vi "setupScene.vi"(11 "Model File Path":path=path "K:/Google_Drive/3d_Parts/Parts_for_printer/forLabview/yArm.stl") -> (3 "reference out":refnum<vi>)   [LabVIEW 2015]
uses:
  <vilib>/Utility/miscctls.llb/LVRGBAColorTypeDef.ctl
  <vilib>/Utility/miscctls.llb/LV3DPointTypeDef.ctl
  <vilib>/picture/3D Picture Control/Object/Create Object (name).vi
  <vilib>/picture/3D Picture Control/NI_3D Picture Control.lvlib
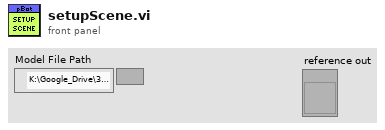
[diagram p1: front panel]
types:
  T1 = enum16{"Inherit Value", "Points", "Wireframe", "Polygons"}
  T2 = typedef "LVRGBAColorTypeDef.ctl" = cluster{"Red":sgl, "Green":sgl, "Blue":sgl, "Alpha":sgl}
  T3 = typedef "LV3DPointTypeDef.ctl" = cluster{"X":sgl, "Y":sgl, "Z":sgl}
  T4 = enum16{"Inherit Value", "Counterclockwise", "Clockwise"}
  T5 = enum16{"Inherit Value", "No Culling", "Cull Back Face", "Cull Front Face", "Cull Both Faces"}
  T6 = enum16{"Normal Bin", "Opaque Bin", "Transparent Bin"}
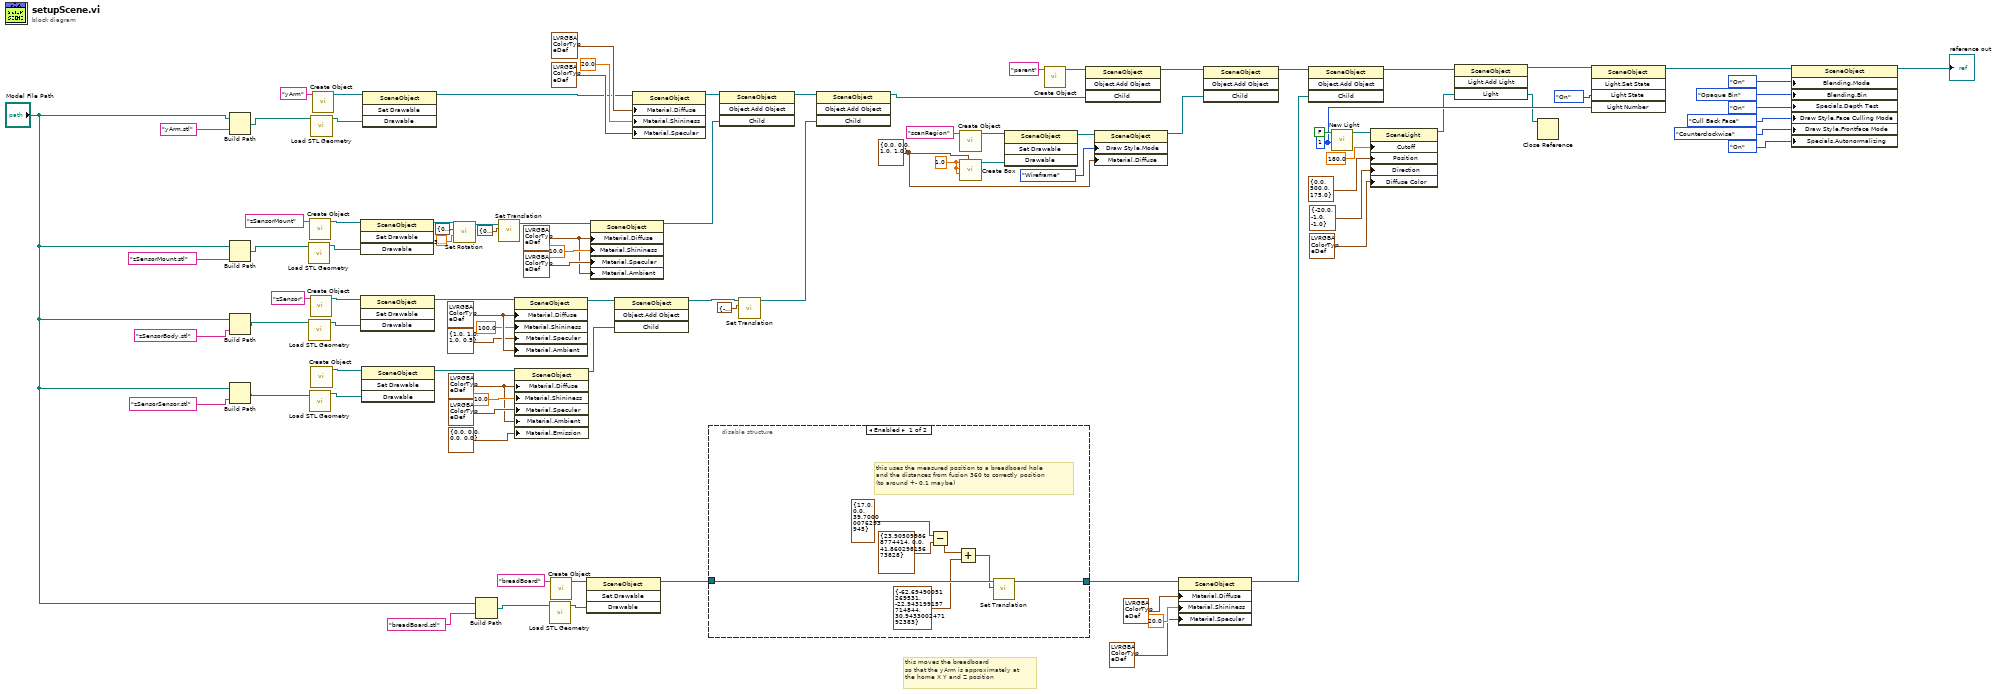
[diagram p0: block diagram]
diagram:
  w4 = T2 {"Red"=0.0, "Green"=0.0, "Blue"=1.0, "Alpha"=1.0} ("Material:Diffuse")
  w8 = sgl 1.0 ("Length X")
  w32 = T2 {"Red"=0.8, "Green"=0.5, "Blue"=0.2, "Alpha"=1.0} ("Material:Specular")
  w43 = T2 {"Red"=0.6, "Green"=0.6, "Blue"=0.6, "Alpha"=1.0} ("Material:Specular")
  w44 = T2 {"Red"=0.7, "Green"=0.7, "Blue"=0.0, "Alpha"=0.9} ("Material:Specular")
  w69 = 1 ("Light Number")
  # "this moves the breadboard\nso that the yArm is approximately at\nthe home X Y and Z position"
  n1 = Build Path(base path="Model File Path", name or relative path="yArm.stl" ("Model File")) -> (appended path=w22:path)
  n2 = Build Path(base path="Model File Path", name or relative path="zSensorMount.stl" ("Model File")) -> (appended path=w16:path)
  n3 = Build Path(base path="Model File Path", name or relative path="zSensorBody.stl" ("Model File")) -> (appended path=w17:path)
  n4 = Build Path(base path="Model File Path", name or relative path="zSensorSensor.stl" ("Model File")) -> (appended path=w18:path)
  n5 = call <vilib>:"Load STL Geometry.vi"("Model File"=w16) -> ("New Mesh Refnum"=w54:refnum<vi>)  [unwired: 9 in, 1 out]
  n6 = call <vilib>:"Load STL Geometry.vi"("Model File"=w17) -> ("New Mesh Refnum"=w40:refnum<vi>)  [unwired: 9 in, 1 out]
  n7 = call-poly <vilib>:"Create Object.vi"("Name"="zSensorMount") -> ("Scene:New Object"=w55:refnum<vi>)  [unwired: 9 in, 1 out]
  n8 = call <vilib>:"Load STL Geometry.vi"("Model File"=w18) -> ("New Mesh Refnum"=w35:refnum<vi>)  [unwired: 9 in, 1 out]
  n9 = call-poly <vilib>:"Create Object.vi"("Name"="zSensor") -> ("Scene:New Object"=w39:refnum<vi>)  [unwired: 9 in, 1 out]
  n10 = call <vilib>:"Load STL Geometry.vi"("Model File"=w22) -> ("New Mesh Refnum"=w93:refnum<vi>)  [unwired: 9 in, 1 out]
  n11 = call-poly <vilib>:"Create Object.vi"() -> ("Scene:New Object"=w36:refnum<vi>)  [unwired: 10 in, 1 out]
  n12 = call-poly <vilib>:"Create Object.vi"("Name"="yArm") -> ("Scene:New Object"=w94:refnum<vi>)  [unwired: 9 in, 1 out]
  n13 = invoke class="SceneObject" method="Set Drawable"(reference=w55, "Drawable"=w54) -> (reference out=w48:refnum<vi>)  [unwired: 2 in, 3 out]
  n14 = invoke class="SceneObject" method="Set Drawable"(reference=w39, "Drawable"=w40) -> (reference out=w30:refnum<vi>)  [unwired: 2 in, 3 out]
  n15 = invoke class="SceneObject" method="Set Drawable"(reference=w36, "Drawable"=w35) -> (reference out=w29:refnum<vi>)  [unwired: 2 in, 3 out]
  n16 = invoke class="SceneObject" method="Set Drawable"(reference=w94, "Drawable"=w93) -> (reference out=w12:refnum<vi>)  [unwired: 2 in, 3 out]
  n17 = call <vilib>:"Set Rotation.vi"("Angle"=3.141592653589793, "Axis"=cluster{"X":sgl, "Y":sgl, "Z":sgl} {"X"=0.0, "Y"=1.0, "Z"=0.0}, "Scene Object"=w48) -> ("Rotated Scene Object"=w45:refnum<vi>)  [unwired: 7 in, 1 out]
  n18 = Build Path(base path="Model File Path", name or relative path="breadBoard.stl" ("Model File")) -> (appended path=w15:path)
  n19 = call <vilib>:"Set Translation.vi"("Translation"=cluster{"X":sgl, "Y":sgl, "Z":sgl} {"X"=0.0, "Y"=4.7625, "Z"=-5.0}, "Scene Object"=w45) -> ("Translated Object"=w51:refnum<vi>)  [unwired: 8 in, 1 out]
  n20 = property class="SceneObject"(reference=w30, "Material.Diffuse"=w43, "Material.Shininess"=sgl 100.0 ("Material:Shininess"), "Material.Specular"=T2 {"Red"=1.0, "Green"=1.0, "Blue"=1.0, "Alpha"=0.5} ("Material:Specular"), "Material.Ambient"=w43) -> (reference out=w37:refnum<vi>)  [unwired: 1 in, 1 out]
  n21 = property class="SceneObject"(reference=w29, "Material.Diffuse"=w32, "Material.Shininess"=sgl 10.0 ("Material:Shininess"), "Material.Specular"=T2 {"Red"=0.5, "Green"=0.2, "Blue"=0.0, "Alpha"=0.5} ("Material:Specular"), "Material.Ambient"=w32, "Material.Emission"=T2 {"Red"=0.0, "Green"=0.0, "Blue"=0.0, "Alpha"=0.0} ("Material:Emission")) -> (reference out=w28:refnum<vi>)  [unwired: 1 in, 1 out]
  n22 = call <vilib>:"Load STL Geometry.vi"("Model File"=w15) -> ("New Mesh Refnum"=w87:refnum<vi>)  [unwired: 9 in, 1 out]
  n23 = call-poly <vilib>:"Create Object.vi"("Name"="breadBoard") -> ("Scene:New Object"=w86:refnum<vi>)  [unwired: 9 in, 1 out]
  n24 = invoke class="SceneObject" method="Set Drawable"(reference=w86, "Drawable"=w87) -> (reference out=w85:refnum<vi>)  [unwired: 2 in, 3 out]
  n25 = property class="SceneObject"(reference=w51, "Material.Diffuse"=w44, "Material.Shininess"=sgl 10.0 ("Material:Shininess"), "Material.Specular"=T2 {"Red"=0.6, "Green"=0.6, "Blue"=0.2, "Alpha"=0.5} ("Material:Specular"), "Material.Ambient"=w44) -> (reference out=w49:refnum<vi>)  [unwired: 1 in, 1 out]
  n26 = invoke class="SceneObject" method="Object.Add Object"(reference=w37, "Child"=w28) -> (reference out=w27:refnum<vi>)  [unwired: 2 in, 3 out]
  n27 = property class="SceneObject"(reference=w12, "Material.Diffuse"=T2 {"Red"=0.3, "Green"=0.3, "Blue"=0.3, "Alpha"=1.0} ("Material:Diffuse"), "Material.Shininess"=sgl 20.0 ("Material:Shininess"), "Material.Specular"=T2 {"Red"=0.4, "Green"=0.4, "Blue"=0.4, "Alpha"=0.8} ("Material:Specular")) -> (reference out=w50:refnum<vi>)  [unwired: 1 in, 1 out]
  n28 = disable-structure shown="Enabled" {
    disable-tunnel: w85 -> [w101 w102]
    disable-tunnel: [w100 w102] -> w74
    frame Enabled {
      # "this uses the measured position to a breadboard hole\nand the distances from fusion 360 to correctly position\n(to around +- 0.1 maybe)"
      n29 = Subtract(x=cluster{"X":sgl, "Y":sgl, "Z":sgl} {"X"=17.0, "Y"=0.0, "Z"=39.7} ("Translation"), y=cluster{"X":sgl, "Y":sgl, "Z":sgl} {"X"=23.9051, "Y"=0.0, "Z"=41.8603} ("Translation")) -> (x-y=w96:cluster{"X":sgl, "Y":sgl, "Z":sgl})
      n30 = Add(x=w96, y=cluster{"X":sgl, "Y":sgl, "Z":sgl} {"X"=-62.6949, "Y"=-22.9432, "Z"=30.9433} ("Translation")) -> (x+y=w95:cluster{"X":sgl, "Y":sgl, "Z":sgl})
      n31 = call <vilib>:"Set Translation.vi"("Translation"=w95, "Scene Object"=w101) -> ("Translated Object"=w100:refnum<vi>)  [unwired: 8 in, 1 out]
    }
    frame Disabled {
    }
  }
  n32 = invoke class="SceneObject" method="Object.Add Object"(reference=w50, "Child"=w49) -> (reference out=w26:refnum<vi>)  [unwired: 2 in, 3 out]
  n33 = call <vilib>:"Set Translation.vi"("Translation"=cluster{"X":sgl, "Y":sgl, "Z":sgl} {"X"=-15.08, "Y"=1.0, "Z"=-5.0}, "Scene Object"=w27) -> ("Translated Object"=w25:refnum<vi>)  [unwired: 8 in, 1 out]
  n34 = invoke class="SceneObject" method="Object.Add Object"(reference=w26, "Child"=w25) -> (reference out=w11:refnum<vi>)  [unwired: 2 in, 3 out]
  n35 = call-poly <vilib>:"Create Object.vi"("Name"="scanRegion") -> ("Scene:New Object"=w6:refnum<vi>)  [unwired: 9 in, 1 out]
  n36 = call <vilib>:"Create Box.vi"("Color"=w4, "Length Z"=w8, "Length Y"=w8, "Length X"=w8) -> ("New Box Refnum"=w1:refnum<vi>)  [unwired: 6 in, 1 out]
  n37 = invoke class="SceneObject" method="Set Drawable"(reference=w6, "Drawable"=w1) -> (reference out=w5:refnum<vi>)  [unwired: 2 in, 3 out]
  n38 = call-poly <vilib>:"Create Object.vi"("Name"="parent") -> ("Scene:New Object"=w91:refnum<vi>)  [unwired: 9 in, 1 out]
  n39 = invoke class="SceneObject" method="Object.Add Object"(reference=w91, "Child"=w11) -> (reference out=w10:refnum<vi>)  [unwired: 2 in, 3 out]
  n40 = property class="SceneObject"(reference=w5, "Draw Style.Mode"=T1."Wireframe" ("Draw Style:Mode"), "Material.Diffuse"=w4) -> (reference out=w2:refnum<vi>)  [unwired: 1 in, 1 out]
  n41 = property class="SceneObject"(reference=w74, "Material.Diffuse"=T2 {"Red"=0.3, "Green"=0.3, "Blue"=0.3, "Alpha"=1.0} ("Material:Diffuse"), "Material.Shininess"=sgl 20.0 ("Material:Shininess"), "Material.Specular"=T2 {"Red"=0.4, "Green"=0.4, "Blue"=0.4, "Alpha"=0.8} ("Material:Specular")) -> (reference out=w73:refnum<vi>)  [unwired: 1 in, 1 out]
  n42 = invoke class="SceneObject" method="Object.Add Object"(reference=w10, "Child"=w2) -> (reference out=w9:refnum<vi>)  [unwired: 2 in, 3 out]
  n43 = invoke class="SceneObject" method="Object.Add Object"(reference=w9, "Child"=w73) -> (reference out=w66:refnum<vi>)  [unwired: 2 in, 3 out]
  n44 = call <vilib>:"New Light.vi"("Light Number"=w69, "At Infinity"=FALSE) -> ("New Light Refnum"=w68:refnum<vi>)  [unwired: 8 in, 1 out]
  n45 = property class="SceneLight"(reference=w68, "Cutoff"=sgl 180.0, "Position"=T3 {"X"=0.0, "Y"=500.0, "Z"=175.0}, "Direction"=T3 {"X"=-20.0, "Y"=-1.0, "Z"=-1.0}, "Diffuse Color"=T2 {"Red"=0.8, "Green"=0.8, "Blue"=1.0, "Alpha"=1.0}) -> (reference out=w65:refnum<vi>)  [unwired: 1 in, 1 out]
  n46 = invoke class="SceneObject" method="Light.Add Light"(reference=w66, "Light"=w65) -> (reference out=w64:refnum<vi>, "Light"=w63:refnum<vi>)  [unwired: 2 in, 2 out]
  n47 = Close Reference(reference=w63) -> ()  [unwired: 1 in, 1 out]
  n48 = invoke class="SceneObject" method="Light.Set State"(reference=w64, "Light State"=enum16{"Inherit Value", "Off", "On"}."On", "Light Number"=w69) -> (reference out=w71:refnum<vi>)  [unwired: 2 in, 4 out]
  n49 = property class="SceneObject"(reference=w71, "Blending.Mode"=enum16{"Inherit Value", "Off", "On"}."On" ("Blending:Mode"), "Blending.Bin"=T6."Opaque Bin" ("Blending:Bin"), "Specials.Depth Test"=enum16{"Inherit Value", "Off", "On"}."On" ("Specials:Depth Test"), "Draw Style.Face Culling Mode"=T5."Cull Back Face" ("Draw Style:Face Culling Mode"), "Draw Style.Frontface Mode"=T4."Counterclockwise" ("Draw Style:Frontface Mode"), "Specials.Autonormalizing"=enum16{"Inherit Value", "Off", "On"}."On" ("Specials:Autonormalizing")) -> (reference out=→"reference out":refnum<vi>)  [unwired: 1 in, 1 out]
